vi "Verify Acquisition.vi"(8 "error in (no error)":errorcluster, 11 "CCDCamera in":refnum<class "Simulated_CCD_Camera.lvclass">) -> (0 "error out":errorcluster, 2 "Acquiring":bool, 3 "CCDCamera out":refnum<class "Simulated_CCD_Camera.lvclass">)   [LabVIEW 2018, in "Simulated_CCD_Camera.lvclass"]
uses:
  Simulated_CCD_Camera.lvclass
  Simulated_CCD_Camera.lvclass/Simulated_CCD_Camera.ctl
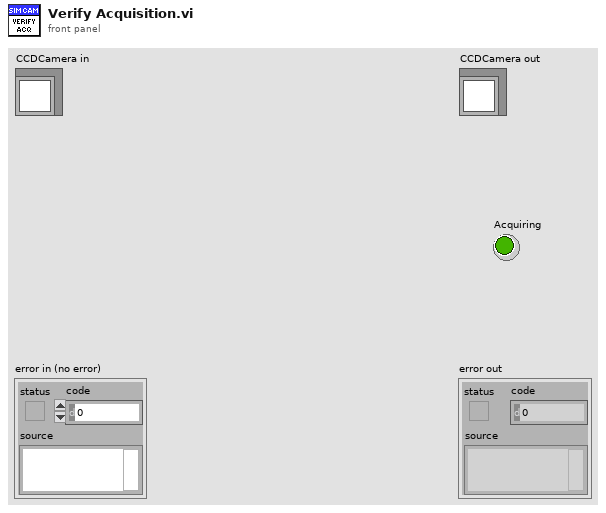
[diagram p1: front panel]
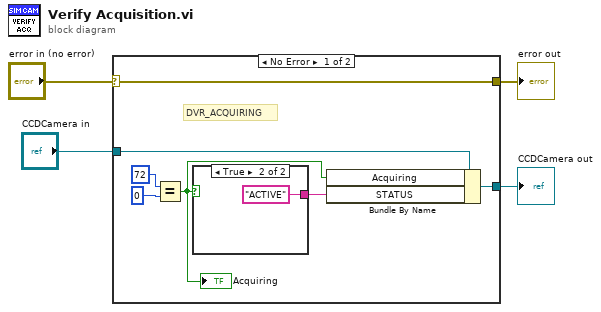
[diagram p0: block diagram]
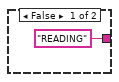
[diagram p2: hidden frame]
diagram:
  n1 = case shown="No Error" "error in (no error)" {
    selector: "error in (no error)" -> [w11 w15]
    tunnel: [w11 w15] -> w3
    tunnel: [w9 w14] -> w1
    tunnel: "CCDCamera in" -> [w10 w14]
    frame No Error {
      # "DVR_ACQUIRING"
      n2 = Equal?(x=72, y=0) -> (x = y?=w8:bool)
      "Acquiring" <- w8
      n3 = case shown="True" w8 {
        tunnel: ["READING" "ACTIVE"] -> w7
        frame False {
        }
        frame True {
        }
      }
      n4 = Bundle By Name(cluster=w10, "Acquiring"=w8, "STATUS"=w7) -> (w9:refnum<class "Simulated_CCD_Camera.lvclass">)
    }
    frame Error {
    }
  }
  "error out" <- w3
  "CCDCamera out" <- w1
